vi "SMR_LabVIEW_V8.2.vi"() -> ()   [LabVIEW 2025]
uses:
  <vilib>/DAQmx/write.llb/DAQmx Write (Analog DBL 1Chan 1Samp).vi
  <vilib>/DAQmx/read.llb/DAQmx Read (Analog 1D DBL NChan 1Samp).vi
  <vilib>/DAQmx/read.llb/DAQmx Read (Analog 2D DBL NChan NSamp).vi
  <vilib>/Analysis/baseanly.llb/Mean (DBL).vi
  <vilib>/DAQmx/create/channels.llb/DAQmx Create Channel (AI-Temperature-Thermocouple).vi
  <vilib>/DAQmx/create/channels.llb/DAQmx Create Channel (AI-Voltage-Basic).vi
  <vilib>/DAQmx/create/channels.llb/DAQmx Create Channel (AO-Voltage-Basic).vi
  <vilib>/DAQmx/miscellaneous.llb/DAQmx Fill In Error Info.vi
  <vilib>/DAQmx/configure/timing.llb/DAQmx Timing (Sample Clock).vi
  <vilib>/addons/control/pid/pid.llb/PID (DBL).vi
  <vilib>/measure/maspectr.llb/FFT Power Spectrum and PSD for 1 Chan.vi
  <vilib>/measure/matone.llb/Extract Single Tone Information 1 Chan.vi
  <vilib>/addons/control/pid/NI_PID_pid.lvlib
  <vilib>/Analysis/NI_AALBase.lvlib
  <vilib>/ptbypt/NI_PtbyPt.lvlib
  <vilib>/measure/NI_MAPro.lvlib
panel:
  out "Rod Power (W)":dbl
  out "Current Through Rod (A)":dbl
  out "Time in Steady State (s)":dbl
  in  "Steady-State Dwell (s)":dbl
  out "Main Loop Flow (GPM)":dbl
  out "FM Amplitude":dbl
  out "FM Frequency":dbl
  out "Spectrum":cluster{"f0":dbl, "df":dbl, "magnitude":dbl[]}(graph)
  out "Raw Signal":waveform(dbl)(graph)
  out "Smoothed HX Flow (GPM)":dbl
  out "Flow History":dbl(graph)
  out "HX Flow (GPM)":dbl
  out "Voltage Across Rod (V)":dbl format="%0.2f"
  out "Current Run Folder":path
  in  "Log Root Folder":path=path "C:/Users/LocalUser/Documents/GitHub/thermal-loop/resources/v0.1.1/data/001"
  out "Raw NI9201 \nVoltage Display":T1
  in  "Loop Period (ms)":dbl=1000.0
  in  "Stop":bool
  out "Auto Steady State Threshold (deg C/min)":dbl
  out "Max dT/dt (deg C/min)":dbl
  out "Temp Change Rate (deg C/min)":dbl
  out "5-Min Baseline Complete":bool
  out "Rate Window Ready":bool
  out "Steady State":bool
  in  "Voltage Limit (V)":dbl=10.0
  in  "Temperature Limit (C)":dbl=50.0
  in  "Pressure Limit (psi)":dbl=15.0
  out "Max Voltage":bool
  out "Max Temperature":bool
  out "Max Pressure":bool
  out "Heat Exchanger Pressure History":dbl(graph)
  out "Main Loop Pressure History":T2(graph)
  out "Overall Avg Pressure (psi)":dbl
  out "Heat Exchanger Pressure P6 (psi)":dbl
  out "Main Loop Avg Pressure (psi)":dbl
  out "Pressure Display":T3
  out "Overall Pressure History":T4(graph)
  out "Max Loop Pressure (psi)":dbl
  out "Heat Exchanger Temperature History":cluster{"Waveform":dbl, "Waveform":dbl}(graph)
  out "Main Loop Temeperature History":T5(graph)
  out "Heat Exchanger Avg Temp (deg C)":dbl
  out "Temperature Display":T6
  out "Overall Temperature History":T7(graph)
  out "Overall Avg Temp (deg C)":dbl
  out "Max Loop Temp (deg C)":dbl
  out "Final P-Valve Voltage (V)":dbl
  out "PID Trim Voltage (V)":dbl
  in  "PID Temp Setpoint (deg C)":dbl
  in  "Auto PID Enable":bool
  in  "Manual P-Valve Voltage (V)":dbl min=0.0 max=10.0
  out "Main Loop Avg Temp (deg C)":dbl
  # "Heat Exchanger Flow"
  # "Control/Troubleshoot"
  # "Steady State"
  # "Emergency Indicators"
  # "Pressure"
  # "Temperature"
  # "Proportional Valve Control"
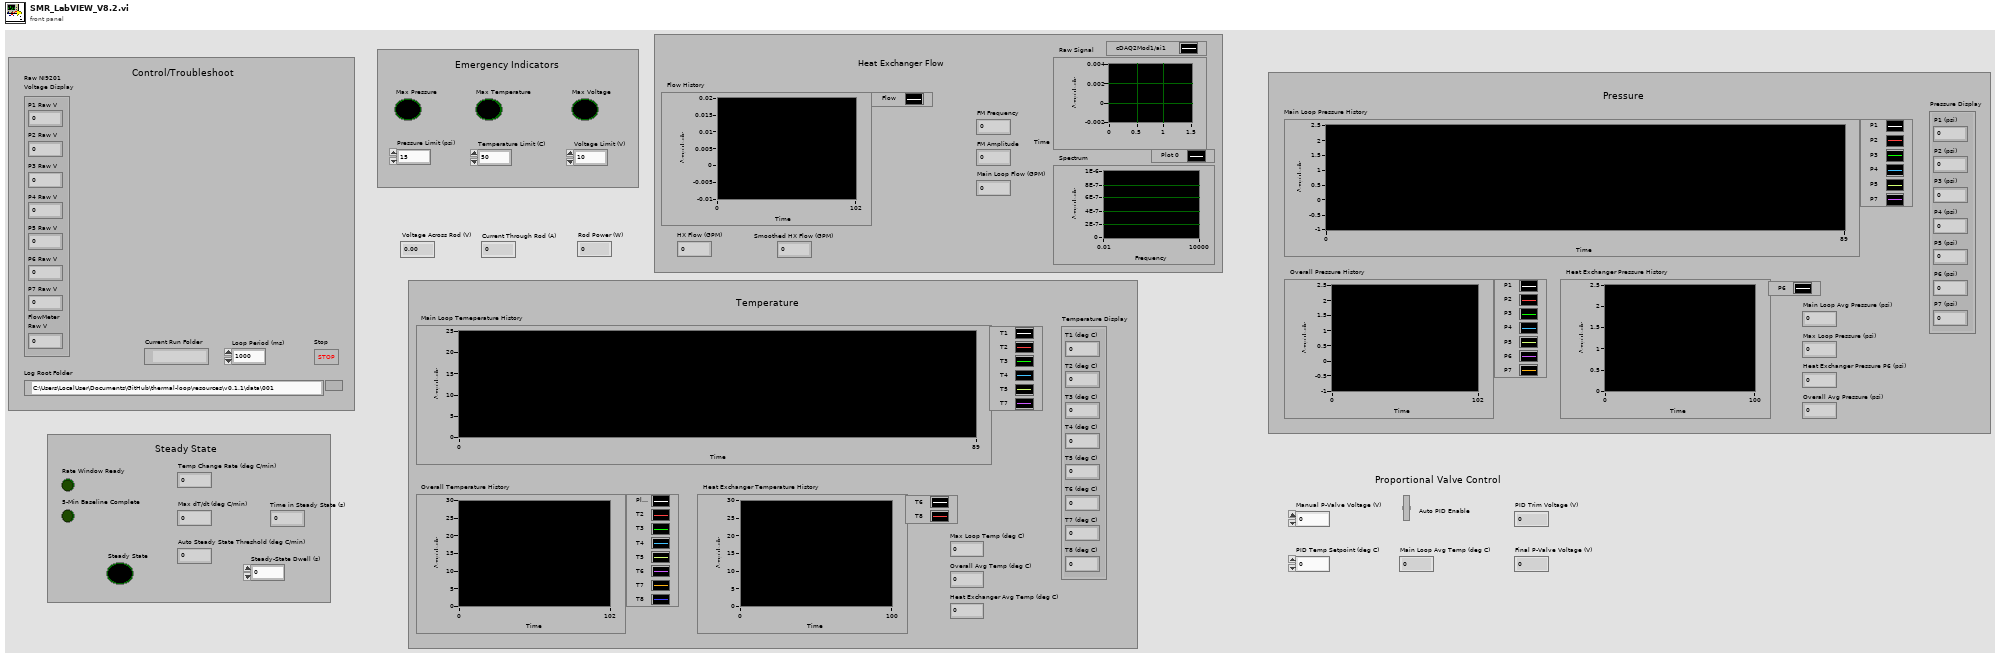
[diagram p1: front panel]
types:
  T1 = cluster{"P1 Raw V":dbl, "P2 Raw V":dbl, "P3 Raw V":dbl, "P4 Raw V":dbl, "P5 Raw V":dbl, "P6 Raw V":dbl, "P7 Raw V":dbl, "FlowMeter\nRaw V":dbl}
  T2 = cluster{"P1":dbl, "P2":dbl, "P3":dbl, "P4":dbl, "P5":dbl, "P7":dbl}
  T3 = cluster{"P1 (psi)":dbl, "P2 (psi)":dbl, "P3 (psi)":dbl, "P4 (psi)":dbl, "P5 (psi)":dbl, "P6 (psi)":dbl, "P7 (psi)":dbl}
  T4 = cluster{"P1":dbl, "P2":dbl, "P3":dbl, "P4":dbl, "P5":dbl, "P6":dbl, "P7":dbl}
  T5 = cluster{"Waveform":dbl, "Waveform":dbl, "Waveform":dbl, "Waveform":dbl, "Waveform":dbl, "Waveform":dbl}
  T6 = cluster{"T1 (deg C)":dbl, "T2 (deg C)":dbl, "T3 (deg C)":dbl, "T4 (deg C)":dbl, "T5 (deg C)":dbl, "T6 (deg C)":dbl, "T7 (deg C)":dbl, "T8 (deg C)":dbl}
  T7 = cluster{"Waveform":dbl, "Waveform":dbl, "Waveform":dbl, "Waveform":dbl, "Waveform":dbl, "Waveform":dbl, "Waveform":dbl, "Waveform":dbl}
  T8 = enum16{"open", "replace", "create", "open or create", "replace or create", "replace or create with confirmation"}
  T9 = cluster{"proportional gain (Kc)":dbl, "integral time (Ti, min)":dbl, "derivative time (Td, min)":dbl}
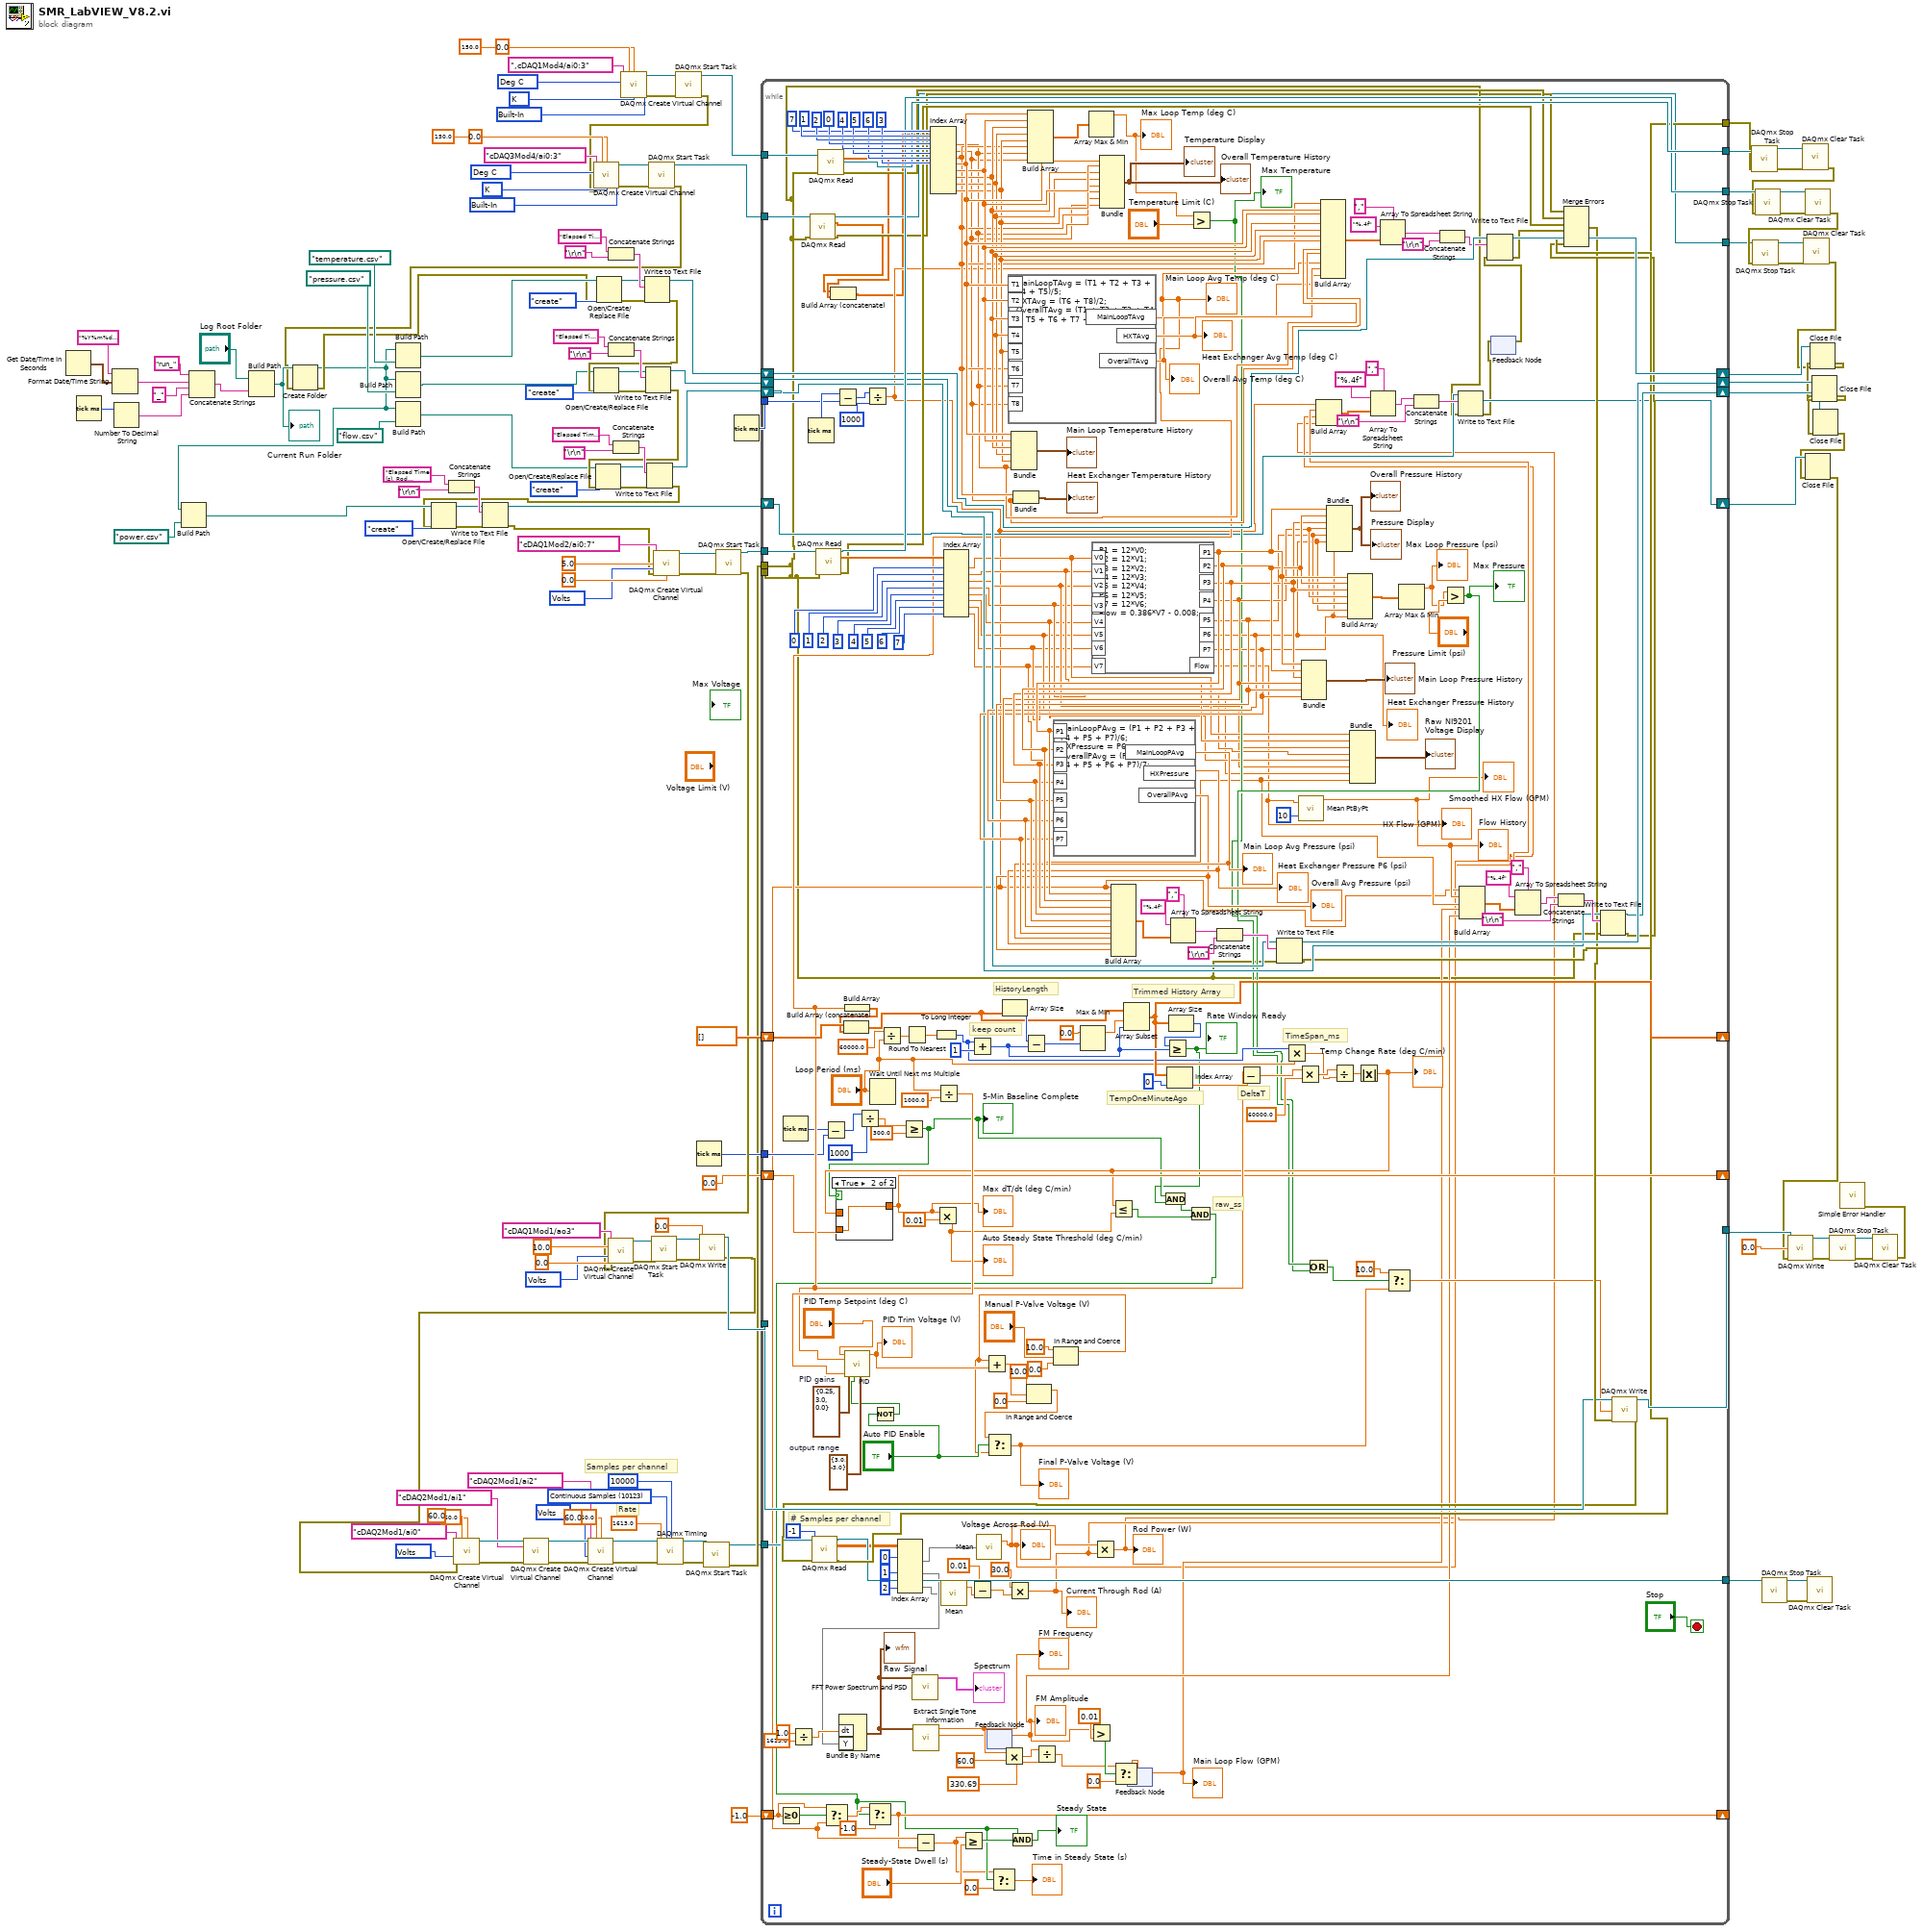
[diagram p0: block diagram]
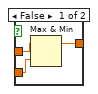
[diagram p2: hidden frame]
diagram:
  w3 = 10348 items=["Volts"=10348, "From Custom Scale"=10065] ("units")
  w20 = 10200 items=["Built-In"=10200, "Constant Value"=10116, "Channel"=10113] ("cjc source")
  w21 = 10073 items=["J"=10072, "K"=10073, "N"=10077, "R"=10082, "S"=10085, "T"=10086, "B"=10047, "E"=10055] ("thermocouple type")
  w22 = 10143 items=["Deg C"=10143, "Deg F"=10144, "Kelvins"=10325, "Deg R"=10145, "From Custom Scale"=10065] ("units")
  w53 = 10123 items=["Finite Samples"=10178, "Continuous Samples"=10123, "Hardware Timed Single Point"=12522] ("sample mode")
  w55 = 10348 items=["Volts"=10348, "From Custom Scale"=10065] ("units")
  w75 = 10348 items=["Volts"=10348, "From Custom Scale"=10065] ("units")
  w137 = 10200 items=["Built-In"=10200, "Constant Value"=10116, "Channel"=10113] ("cjc source")
  w138 = 10073 items=["J"=10072, "K"=10073, "N"=10077, "R"=10082, "S"=10085, "T"=10086, "B"=10047, "E"=10055] ("thermocouple type")
  w139 = 10143 items=["Deg C"=10143, "Deg F"=10144, "Kelvins"=10325, "Deg R"=10145, "From Custom Scale"=10065] ("units")
  w146 = 10348 items=["Volts"=10348, "From Custom Scale"=10065] ("units")
  # "Samples per channel"
  # "Rate"
  n1 = Get Date/Time In Seconds() -> (seconds since 1Jan1904=w96:timestamp)
  n2 = Tick Count (ms)() -> (millisecond timer value=w94:u32)
  n3 = Format Date/Time String(time format string (%c)="%Y%m%d_%H%M%S", seconds (now)=w96) -> (date/time string=w91:string)  [unwired: 1 in]
  n4 = Number To Decimal String(number=w94) -> (decimal integer string=w92:string)  [unwired: 1 in]
  n5 = Concatenate Strings("run_" ("string"), w91, "_" ("string"), w92) -> (w88:string)
  n6 = Build Path(base path="Log Root Folder", name or relative path=w88) -> (appended path=w87:path)
  "Current Run Folder" <- w87
  n7 = Concatenate Strings("Elapsed Time (s), Rod voltage (V), Rod Current (A), Rod Power (W)", "\r\n") -> (w39:string)
  n8 = Concatenate Strings("Elapsed Time (s),T1 (deg C),T2 (deg C),T3 (deg C),T4 (deg C),T5 (deg C),T6 (deg C),T7 (deg C),T8 (deg C),Main Loop Avg Temp (deg C),HX Avg Temp (deg C),Overall Avg Temp (deg C)", "\r\n") -> (w120:string)
  n9 = Concatenate Strings("Elapsed Time (s),P1 (psi),P2 (psi),P3 (psi),P4 (psi),P5 (psi),P6 (psi),P7 (psi),Main Loop Avg Pressure (psi),HX Pressure (psi),Overall Avg Pressure (psi)", "\r\n") -> (w118:string)
  n10 = Concatenate Strings("Elapsed Time (s),Heat Exchanger Flow (GPM),Flow Raw Voltage (V), Main Loop Flow (GPM), Flow Signal Amplitude (V)", "\r\n") -> (w114:string)
  n11 = call-poly <vilib>:"DAQmx Create Virtual Channel.vi"("maximum value"=150.0, "minimum value"=0.0, "physical channels"=tag ",cDAQ1Mod4/ai0:3", "cjc source"=w137, "units"=w139, "thermocouple type"=w138) -> ("task out"=w136:refnum<k21>, "error out"=w135:errorcluster)  [unwired: 8 in]
  n12 = call <vilib>:"DAQmx Start Task.vi"("task/channels in"=w136, "error in"=w135) -> ("task out"=w134:refnum<k21>, "error out"=w16:errorcluster)  [unwired: 12 in]
  n13 = call-poly <vilib>:"DAQmx Create Virtual Channel.vi"("maximum value"=150.0, "minimum value"=0.0, "physical channels"=tag "cDAQ3Mod4/ai0:3", "cjc source"=w20, "units"=w22, "error in"=w16, "thermocouple type"=w21) -> ("task out"=w19:refnum<k21>, "error out"=w18:errorcluster)  [unwired: 7 in]
  n14 = call <vilib>:"DAQmx Start Task.vi"("task/channels in"=w19, "error in"=w18) -> ("task out"=w14:refnum<k21>, "error out"=w15:errorcluster)  [unwired: 12 in]
  n15 = Create Folder(path (use dialog)=w87, error in=w15) -> (created path=w33:path, error out=w80:errorcluster)  [unwired: 1 in, 1 out]
  n16 = Build Path(base path=w33, name or relative path=path "power.csv") -> (appended path=w34:path)
  n17 = Build Path(base path=w33, name or relative path=path "temperature.csv") -> (appended path=w86:path)
  n18 = Build Path(base path=w33, name or relative path=path "pressure.csv") -> (appended path=w85:path)
  n19 = Build Path(base path=w33, name or relative path=path "flow.csv") -> (appended path=w84:path)
  n20 = Open/Create/Replace File(file path (use dialog)=w86, error in=w80, operation (0:open)=T8."create") -> (refnum out=w119:refnum<file>, error out=w103:errorcluster)  [unwired: 3 in, 1 out]
  n21 = Write to Text File(file (use dialog)=w119, text=w120, error in=w103) -> (refnum out=w110:refnum<file>, error out=w102:errorcluster)  [unwired: 1 in, 1 out]
  n22 = Open/Create/Replace File(file path (use dialog)=w85, error in=w102, operation (0:open)=T8."create") -> (refnum out=w117:refnum<file>, error out=w101:errorcluster)  [unwired: 3 in, 1 out]
  n23 = Write to Text File(file (use dialog)=w117, text=w118, error in=w101) -> (refnum out=w109:refnum<file>, error out=w100:errorcluster)  [unwired: 1 in, 1 out]
  n24 = Open/Create/Replace File(file path (use dialog)=w84, error in=w100, operation (0:open)=T8."create") -> (refnum out=w113:refnum<file>, error out=w99:errorcluster)  [unwired: 3 in, 1 out]
  n25 = Write to Text File(file (use dialog)=w113, text=w114, error in=w99) -> (refnum out=w108:refnum<file>, error out=w31:errorcluster)  [unwired: 1 in, 1 out]
  n26 = Open/Create/Replace File(file path (use dialog)=w34, error in=w31, operation (0:open)=T8."create") -> (refnum out=w38:refnum<file>, error out=w35:errorcluster)  [unwired: 3 in, 1 out]
  n27 = Write to Text File(file (use dialog)=w38, text=w39, error in=w35) -> (refnum out=w29:refnum<file>, error out=w30:errorcluster)  [unwired: 1 in, 1 out]
  n28 = call-poly <vilib>:"DAQmx Create Virtual Channel.vi"("maximum value"=5.0, "minimum value"=0.0, "physical channels"=tag "cDAQ1Mod2/ai0:7", "units"=w146, "error in"=w30) -> ("task out"=w145:refnum<k21>, "error out"=w144:errorcluster)  [unwired: 9 in]
  n29 = Tick Count (ms)() -> (millisecond timer value=w60:u32)
  n30 = call <vilib>:"DAQmx Start Task.vi"("task/channels in"=w145, "error in"=w144) -> ("task out"=w143:refnum<k21>, "error out"=w68:errorcluster)  [unwired: 12 in]
  n31 = call-poly <vilib>:"DAQmx Create Virtual Channel.vi"("maximum value"=10.0, "minimum value"=0.0, "physical channels"=tag "cDAQ1Mod1/ao3", "units"=w75, "error in"=w68) -> ("task out"=w74:refnum<k21>, "error out"=w73:errorcluster)  [unwired: 9 in]
  n32 = call <vilib>:"DAQmx Start Task.vi"("task/channels in"=w74, "error in"=w73) -> ("task out"=w72:refnum<k21>, "error out"=w71:errorcluster)  [unwired: 12 in]
  n33 = call-poly <vilib>:"DAQmx Write.vi"("task/channels in"=w72, "data"=0.0, "error in"=w71) -> ("task out"=w69:refnum<k21>, "error out"=w47:errorcluster)  [unwired: 10 in, 1 out]
  n34 = call-poly <vilib>:"DAQmx Create Virtual Channel.vi"("maximum value"=60.0, "minimum value"=-60.0, "physical channels"=tag "cDAQ2Mod1/ai0", "units"=w55, "error in"=w47) -> ("task out"=w43:refnum<k21>, "error out"=w42:errorcluster)  [unwired: 9 in]
  n35 = call-poly <vilib>:"DAQmx Create Virtual Channel.vi"("task in"=w43, "physical channels"=tag "cDAQ2Mod1/ai1", "error in"=w42) -> ("task out"=w7:refnum<k21>, "error out"=w5:errorcluster)  [unwired: 11 in]
  n36 = call-poly <vilib>:"DAQmx Create Virtual Channel.vi"("task in"=w7, "maximum value"=60.0, "minimum value"=-60.0, "physical channels"=tag "cDAQ2Mod1/ai2", "units"=w3, "error in"=w5) -> ("task out"=w6:refnum<k21>, "error out"=w4:errorcluster)  [unwired: 8 in]
  n37 = call-poly <vilib>:"DAQmx Timing.vi"("task/channels in"=w6, "sample mode"=w53, "samples per channel"=10000, "rate"=1613.0, "error in"=w4) -> ("task out"=w51:refnum<k21>, "error out"=w50:errorcluster)  [unwired: 9 in]
  n38 = call <vilib>:"DAQmx Start Task.vi"("task/channels in"=w51, "error in"=w50) -> ("task out"=w45:refnum<k21>, "error out"=w46:errorcluster)  [unwired: 12 in]
  n39 = Tick Count (ms)() -> (millisecond timer value=w107:u32)
  n40 = while {
    tunnel: w143 -> [w375]
    tunnel: w134 -> [w358]
    tunnel: [w349] -> w133
    tunnel: [w164] -> _
    tunnel: [w348] -> w132
    tunnel: [w224] -> w131
    shift-right: [w325] -> w106
    shift-left: w110 -> [w326]
    shift-right: [w306] -> w105
    shift-left: w109 -> [w307]
    shift-right: [w298] -> w104
    shift-left: w108 -> [w299]
    tunnel: w107 -> [w344]
    shift-right: [w277] -> _
    shift-left: dbl[] [] -> [w290]
    tunnel: w69 -> [w258]
    tunnel: w46 -> [w164]
    tunnel: [w265] -> w66
    tunnel: w60 -> [w247]
    shift-right: [w240] -> _
    shift-left: 0.0 -> [w242]
    tunnel: w45 -> [w223]
    tunnel: [w222] -> w44
    shift-right: [w181] -> w28
    shift-left: w29 -> [w182]
    shift-right: [w173] -> _
    shift-left: -1.0 -> [w177]
    tunnel: w14 -> [w165]
    tunnel: [w162] -> w10
    stop <- "Stop" stop-if-true
    w263 = cluster{"output high":dbl, "output low":dbl} {"output high"=3.0, "output low"=-3.0}  # output range
    w264 = T9 {"proportional gain (Kc)"=0.25, "integral time (Ti, min)"=3.0, "derivative time (Td, min)"=0.0}  # PID gains
    # "raw_ss"
    # "# Samples per channel"
    # "TimeSpan_ms"
    # "DeltaT"
    # "TempOneMinuteAgo"
    # "Trimmed History Array"
    # "HistoryLength"
    # "keep count"
    n41 = Greater Or Equal To 0?(x=w177) -> (x >= 0?=w178:bool)
    n42 = Tick Count (ms)() -> (millisecond timer value=w248:u32)
    n43 = Divide(x=1.0, y=1613.0) -> (x/y=w195:dbl)
    n44 = Tick Count (ms)() -> (millisecond timer value=w345:u32)
    n45 = call-poly <vilib>:"DAQmx Read.vi"("task/channels in"=w165, "error in"=w164) -> ("task out"=w162:refnum<k21>, "data"=w159:dbl[], "error out"=w163:errorcluster)  [unwired: 11 in]
    n46 = call-poly <vilib>:"DAQmx Read.vi"("task/channels in"=w375, "error in"=w164) -> ("task out"=w348:refnum<k21>, "data"=w366:dbl[], "error out"=w346:errorcluster)  [unwired: 11 in]
    n47 = call-poly <vilib>:"DAQmx Read.vi"("task/channels in"=w358, "error in"=w164) -> ("task out"=w349:refnum<k21>, "data"=w160:dbl[], "error out"=w347:errorcluster)  [unwired: 11 in]
    n48 = Subtract(x=w248, y=w247) -> (x-y=w246:u32)
    n49 = Build Array (concatenate)(w159, w160) -> (w161:dbl[])
    n50 = Subtract(x=w345, y=w344) -> (x-y=w343:u32)
    n51 = Divide(x=w246, y=u32 1000) -> (x/y=w244:dbl)
    n52 = Divide(x=w343, y=u32 1000) -> (x/y=w174:dbl)
    n53 = Select(t=w177, s=w178, f=w174) -> (s? t:f=w176:dbl)
    n54 = Wait Until Next ms Multiple(millisecond multiple="Loop Period (ms)") -> ()  [unwired: 1 out]
    n55 = Not(x="Auto PID Enable") -> (.not. x?=w259:bool)
    n56 = Divide(x=60000.0, y="Loop Period (ms)") -> (x/y=w287:dbl)
    n57 = Greater Or Equal?(x=w244, y=300.0) -> (x >= y?=w237:bool)
    "5-Min Baseline Complete" <- w237
    n58 = Round To Nearest(number=w287) -> (nearest integer value=w286:dbl)
    n59 = Index Array(array=w161, index #1=7 ("index"), index #2=1 ("index"), index #3=2 ("index"), index #4=0 ("index"), index #5=4 ("index"), index #6=5 ("index"), index #7=6 ("index"), index #8=3 ("index")) -> (element #1=w335:dbl, element #2=w334:dbl, element #3=w336:dbl, element #4=w341:dbl, element #5=w340:dbl, element #6=w339:dbl, element #7=w338:dbl, element #8=w337:dbl)
    n60 = To Long Integer(number=w286) -> (32bit integer=w274:i32)
    n61 = Divide(x="Loop Period (ms)", y=1000.0) -> (x/y=w260:dbl)
    n62 = Index Array(array=w366, index #1=0 ("index"), index #2=1 ("index"), index #3=2 ("index"), index #4=3 ("index"), index #5=4 ("index"), index #6=5 ("index"), index #7=6 ("index"), index #8=7 ("index")) -> (element #1=w221:dbl, element #2=w220:dbl, element #3=w219:dbl, element #4=w218:dbl, element #5=w217:dbl, element #6=w216:dbl, element #7=w215:dbl, element #8=w214:dbl)
    n63 = Add(x=w274, y=1) -> (x+y=w279:i32)
    n64 = feedback #1() -> (w191:dbl)  [unwired: 1 in]
    "FM Amplitude" <- w191
    n65 = formula code="MainLoopTAvg = (T1 + T2 + T3 + T4 + T5)/5;\nHXTAvg = (T6 + T8)/2;\nOverallTAvg = (T1 + T2 + T3 + T4 + T5 + T6 + T7 + T8)/8;"("T1"=w341, "T2"=w340, "T3"=w339, "T4"=w338, "T5"=w337, "T6"=w336, "T7"=w335, "T8"=w334) -> ("MainLoopTAvg"=w250:dbl, "HXTAvg"=w333:dbl, "OverallTAvg"=w332:dbl)
    "Overall Avg Temp (deg C)" <- w332
    "Main Loop Avg Temp (deg C)" <- w250
    "Heat Exchanger Avg Temp (deg C)" <- w333
    n66 = Build Array(w250) -> (w289:dbl[])
    n67 = Build Array (concatenate)(w290, w289) -> (w281:dbl[])
    n68 = call-poly <vilib>:"PID.vi"("reinitialize? (F)"=w259, "output range"=w263, "dt (s)"=w260, "PID gains"=w264, "process variable"=w250, "setpoint"="PID Temp Setpoint (deg C)") -> ("output"=w257:dbl)  [unwired: 4 in, 1 out]
    "PID Trim Voltage (V)" <- w257
    n69 = Array Size(array=w281) -> (size(s)=w284:i32)
    n70 = Bundle("Waveform"=w341, "Waveform"=w340, "Waveform"=w339, "Waveform"=w338, "Waveform"=w337, "Waveform"=w335) -> (→"Main Loop Temeperature History":T5)  [unwired: 1 in]
    n71 = Bundle("Waveform"=w336, "Waveform"=w334) -> (→"Heat Exchanger Temperature History":cluster{"Waveform":dbl, "Waveform":dbl})  [unwired: 1 in]
    n72 = Subtract(x=w284, y=w279) -> (x-y=w282:i32)
    n73 = Build Array(w341, w340, w339, w338, w337, w336, w335, w334) -> (w376:dbl[])
    n74 = In Range and Coerce(upper limit=10.0, x="Manual P-Valve Voltage (V)", lower limit=0.0) -> (coerced(x)=w252:dbl)  [unwired: 1 out]
    n75 = Add(x=w252, y=w257) -> (x+y=w256:dbl)
    n76 = In Range and Coerce(upper limit=10.0, x=w256, lower limit=0.0) -> (coerced(x)=w251:dbl)  [unwired: 1 out]
    n77 = Select(t=w251, s="Auto PID Enable", f=w252) -> (s? t:f=w229:dbl)
    "Final P-Valve Voltage (V)" <- w229
    n78 = Max & Min(x=0.0, y=w282) -> (max(x,y)=w280:dbl)  [unwired: 1 out]
    n79 = Array Max & Min(array=w376) -> (max value=w292:dbl)  [unwired: 3 out]
    "Max Loop Temp (deg C)" <- w292
    n80 = Greater?(x=w191, y=0.01) -> (0:w199:bool)
    n81 = formula code="P1 = 12*V0;\nP2 = 12*V1;\nP3 = 12*V2;\nP4 = 12*V3;\nP5 = 12*V4;\nP6 = 12*V5; \nP7 = 12*V6;\nFlow = 0.386*V7 - 0.008;"("V0"=w221, "V1"=w220, "V2"=w219, "V3"=w218, "V4"=w217, "V5"=w216, "V6"=w215, "V7"=w214) -> ("P1"=w324:dbl, "P2"=w323:dbl, "P3"=w322:dbl, "P4"=w321:dbl, "P5"=w320:dbl, "P6"=w319:dbl, "P7"=w318:dbl, "Flow"=w213:dbl)
    "HX Flow (GPM)" <- w213
    "Heat Exchanger Pressure History" <- w319
    n82 = formula code="MainLoopPAvg = (P1 + P2 + P3 + P4 + P5 + P7)/6;\nHXPressure = P6;\nOverallPAvg = (P1 + P2 + P3 + P4 + P5 + P6 + P7)/7;"("P1"=w324, "P2"=w323, "P3"=w322, "P4"=w321, "P5"=w320, "P6"=w319, "P7"=w318) -> ("MainLoopPAvg"=w317:dbl, "HXPressure"=w316:dbl, "OverallPAvg"=w315:dbl)
    "Overall Avg Pressure (psi)" <- w315
    "Heat Exchanger Pressure P6 (psi)" <- w316
    "Main Loop Avg Pressure (psi)" <- w317
    n83 = Bundle("Waveform"=w341, "Waveform"=w340, "Waveform"=w339, "Waveform"=w338, "Waveform"=w337, "Waveform"=w336, "Waveform"=w335, "Waveform"=w334) -> (→"Overall Temperature History" →"Temperature Display":T7)  [unwired: 1 in]
    n84 = Build Array(w174, w324, w323, w322, w321, w320, w319, w318, w317, w316, w315) -> (w314:dbl[])
    n85 = Array Subset(array=w281, index=w280, length=w279) -> (w277:dbl[])
    n86 = feedback #2() -> (w189:dbl)  [unwired: 1 in]
    "Main Loop Flow (GPM)" <- w189
    n87 = Index Array(array=w277, index=0) -> (element=w275:dbl)
    n88 = Array Size(array=w277) -> (size(s)=w278:i32)
    n89 = Greater Or Equal?(x=w278, y=w279) -> (x >= y?=w236:bool)
    "Rate Window Ready" <- w236
    n90 = And(x=w237, y=w236) -> (x .and. y?=w235:bool)
    n91 = Array To Spreadsheet String(delimiter (Tab)=",", array=w314, 3:"%.4f" ("format string")) -> (spreadsheet string=w310:string)
    n92 = Greater?(x=w292, y="Temperature Limit (C)") -> (0:w232:bool)
    "Max Temperature" <- w232
    n93 = Concatenate Strings(w310, "\r\n") -> (w308:string)
    n94 = Subtract(x=w250, y=w275) -> (x-y=w273:dbl)
    n95 = Write to Text File(file (use dialog)=w307, text=w308, error in=w164) -> (refnum out=w306:refnum<file>, error out=w296:errorcluster)  [unwired: 1 in, 1 out]
    n96 = Multiply(x=w274, y="Loop Period (ms)") -> (x*y=w270:dbl)
    n97 = Multiply(x=w273, y=60000.0) -> (x*y=w271:dbl)
    n98 = call <vilib>:"Mean PtByPt.vi"("x"=w213, "sample length"=10) -> ("mean"=w211:dbl)  [unwired: 2 in, 1 out]
    "Flow History" <- w211
    "Smoothed HX Flow (GPM)" <- w211
    n99 = Bundle("P1"=w324, "P2"=w323, "P3"=w322, "P4"=w321, "P5"=w320, "P7"=w318) -> (→"Main Loop Pressure History":T2)  [unwired: 1 in]
    n100 = Build Array(w174, w341, w340, w339, w338, w337, w336, w335, w334, w250, w333, w332) -> (w331:dbl[])
    n101 = Bundle("P1"=w324, "P2"=w323, "P3"=w322, "P4"=w321, "P5"=w320, "P6"=w319, "P7"=w318) -> (→"Overall Pressure History" →"Pressure Display":T4)  [unwired: 1 in]
    n102 = Divide(x=w271, y=w270) -> (x/y=w269:dbl)
    n103 = Build Array(w324, w323, w322, w321, w320, w319, w318) -> (w365:dbl[])
    n104 = Bundle("Waveform"=w221, "Waveform"=w220, "Waveform"=w219, "Waveform"=w218, "Waveform"=w217, "Waveform"=w216, "Waveform"=w215, "Waveform"=w214) -> (→"Raw NI9201 \nVoltage Display":T7)  [unwired: 1 in]
    n105 = Absolute Value(x=w269) -> (abs(x)=w239:dbl)
    "Temp Change Rate (deg C/min)" <- w239
    n106 = case shown="True" w237 {
      tunnel: w242 -> [w380 w381]
      tunnel: w239 -> [w379 _]
      tunnel: [w378 w381] -> w240
      frame False {
        n107 = Max & Min(x=w379, y=w380) -> (max(x,y)=w378:dbl)  [unwired: 1 out]
      }
      frame True {
      }
    }
    "Max dT/dt (deg C/min)" <- w240
    n108 = Multiply(x=w240, y=0.01) -> (x*y=w238:dbl)
    "Auto Steady State Threshold (deg C/min)" <- w238
    n109 = Less Or Equal?(x=w239, y=w238) -> (x <= y?=w234:bool)
    n110 = And(x=w235, y=w234) -> (x .and. y?=w169:bool)
    n111 = Select(t=w176, s=w169, f=-1.0) -> (s? t:f=w173:dbl)
    n112 = Subtract(x=w174, y=w173) -> (x-y=w168:dbl)
    n113 = Greater Or Equal?(x=w168, y="Steady-State Dwell (s)") -> (x >= y?=w171:bool)
    n114 = Select(t=w168, s=w169, f=0.0) -> (s? t:f=→"Time in Steady State (s)":dbl)
    n115 = And(x=w169, y=w171) -> (x .and. y?=→"Steady State":bool)
    n116 = Array To Spreadsheet String(delimiter (Tab)=",", array=w331, 3:"%.4f" ("format string")) -> (spreadsheet string=w328:string)
    n117 = Array Max & Min(array=w365) -> (max value=w293:dbl)  [unwired: 3 out]
    "Max Loop Pressure (psi)" <- w293
    n118 = Concatenate Strings(w328, "\r\n") -> (w311:string)
    n119 = Greater?(x=w293, y="Pressure Limit (psi)") -> (0:w233:bool)
    "Max Pressure" <- w233
    n120 = Or(x=w233, y=w232) -> (x .or. y?=w227:bool)
    n121 = Select(t=10.0, s=w227, f=w229) -> (s? t:f=w228:dbl)
    n122 = Build Array(w174, w211, w214, w189, w191) -> (w305:dbl[])
    n123 = feedback #3() -> (w179:errorcluster)  [unwired: 1 in]
    n124 = Write to Text File(file (use dialog)=w326, text=w311, error in=w179) -> (refnum out=w325:refnum<file>, error out=w297:errorcluster)  [unwired: 1 in, 1 out]
    n125 = Array To Spreadsheet String(delimiter (Tab)=",", array=w305, 3:"%.4f" ("format string")) -> (spreadsheet string=w301:string)
    n126 = Concatenate Strings(w301, "\r\n") -> (w300:string)
    n127 = Write to Text File(file (use dialog)=w299, text=w300, error in=w164) -> (refnum out=w298:refnum<file>, error out=w295:errorcluster)  [unwired: 1 in, 1 out]
    n128 = Merge Errors(w163, w347, w346, w297, w296, w295) -> (w266:errorcluster)
    n129 = call-poly <vilib>:"DAQmx Write.vi"("task/channels in"=w258, "data"=w228, "error in"=w266) -> ("task out"=w265:refnum<k21>, "error out"=w225:errorcluster)  [unwired: 10 in, 1 out]
    n130 = call-poly <vilib>:"DAQmx Read.vi"("task/channels in"=w223, "number of samples per channel"=-1, "error in"=w225) -> ("task out"=w222:refnum<k21>, "data"=w210:dbl[][], "error out"=w224:errorcluster)  [unwired: 10 in]
    n131 = Index Array(array=w210, index (row) #1=0 ("index (row)"), index (row) #2=1 ("index (row)"), index (row) #3=2 ("index (row)")) -> (element #1=w209:dbl[], element #2=w194:dbl[], element #3=w154:dbl[])  [unwired: 3 in]
    n132 = Bundle By Name("dt"=w195, "Y"=w194) -> (w193:waveform(dbl))  [unwired: 1 in]
    "Raw Signal" <- w193
    n133 = call-poly <vilib>:"FFT Power Spectrum and PSD.vi"("time signal"=w193) -> ("Power Spectrum / PSD"=→"Spectrum":cluster{"f0":dbl, "df":dbl, "magnitude":dbl[]})  [unwired: 7 in, 3 out]
    n134 = call-poly <vilib>:"Extract Single Tone Information.vi"("time signal in"=w193) -> ("detected amplitude"=w192:dbl, "detected frequency"=w205:dbl)  [unwired: 5 in, 4 out]
    "FM Frequency" <- w205
    n135 = call-poly <vilib>:"Mean.vi"("X"=w154) -> ("mean"=w155:dbl)  [unwired: 1 out]
    n136 = Subtract(x=0.01, y=w155) -> (x-y=w156:dbl)
    n137 = call-poly <vilib>:"Mean.vi"("X"=w209) -> ("mean"=w152:dbl)  [unwired: 1 out]
    "Voltage Across Rod (V)" <- w152
    n138 = feedback-in #1(w192) -> ()
    n139 = Multiply(x=w205, y=60.0) -> (x*y=w203:dbl)
    n140 = Multiply(x=30.0, y=w156) -> (x*y=w151:dbl)
    "Current Through Rod (A)" <- w151
    n141 = Divide(x=w203, y=330.69) -> (x/y=w198:dbl)
    n142 = Multiply(x=w152, y=w151) -> (x*y=w150:dbl)
    "Rod Power (W)" <- w150
    n143 = Select(t=w198, s=w199, f=0.0) -> (s? t:f=w190:dbl)
    n144 = feedback-in #2(w190) -> ()
    n145 = Build Array(w174, w152, w151, w150) -> (w184:dbl[])
    n146 = Array To Spreadsheet String(delimiter (Tab)=",", array=w184, 3:"%.4f" ("format string")) -> (spreadsheet string=w187:string)
    n147 = Concatenate Strings(w187, "\r\n") -> (w183:string)
    n148 = Write to Text File(file (use dialog)=w182, text=w183, error in=w164) -> (refnum out=w181:refnum<file>, error out=w180:errorcluster)  [unwired: 1 in, 1 out]
    n149 = feedback-in #3(w180) -> ()
  }
  n150 = call <vilib>:"DAQmx Stop Task.vi"("task/channels in"=w133, "error in"=w131) -> ("task out"=w130:refnum<k21>, "error out"=w128:errorcluster)  [unwired: 12 in]
  n151 = call <vilib>:"DAQmx Stop Task.vi"("task/channels in"=w44) -> ("task out"=w49:refnum<k21>, "error out"=w48:errorcluster)  [unwired: 13 in]
  n152 = call <vilib>:"DAQmx Clear Task.vi"("task in"=w130, "error in"=w128) -> ("error out"=w127:errorcluster)  [unwired: 13 in]
  n153 = call <vilib>:"DAQmx Stop Task.vi"("task/channels in"=w132, "error in"=w127) -> ("task out"=w129:refnum<k21>, "error out"=w126:errorcluster)  [unwired: 12 in]
  n154 = call <vilib>:"DAQmx Clear Task.vi"("task in"=w129, "error in"=w126) -> ("error out"=w13:errorcluster)  [unwired: 13 in]
  n155 = call <vilib>:"DAQmx Stop Task.vi"("task/channels in"=w10, "error in"=w13) -> ("task out"=w9:refnum<k21>, "error out"=w12:errorcluster)  [unwired: 12 in]
  n156 = call <vilib>:"DAQmx Clear Task.vi"("task in"=w9, "error in"=w12) -> ("error out"=w11:errorcluster)  [unwired: 13 in]
  n157 = call <vilib>:"DAQmx Clear Task.vi"("task in"=w49, "error in"=w48) -> ()  [unwired: 13 in, 1 out]
  n158 = Close File(refnum=w106, error in=w11) -> (error out=w98:errorcluster)  [unwired: 1 out]
  n159 = Close File(refnum=w105, error in=w98) -> (error out=w97:errorcluster)  [unwired: 1 out]
  n160 = Close File(refnum=w104, error in=w97) -> (error out=w27:errorcluster)  [unwired: 1 out]
  n161 = Close File(refnum=w28, error in=w27) -> (error out=w26:errorcluster)  [unwired: 1 out]
  n162 = call-poly <vilib>:"DAQmx Write.vi"("task/channels in"=w66, "data"=0.0, "error in"=w26) -> ("task out"=w65:refnum<k21>, "error out"=w63:errorcluster)  [unwired: 10 in, 1 out]
  n163 = call <vilib>:"DAQmx Stop Task.vi"("task/channels in"=w65, "error in"=w63) -> ("task out"=w64:refnum<k21>, "error out"=w62:errorcluster)  [unwired: 12 in]
  n164 = call <vilib>:"DAQmx Clear Task.vi"("task in"=w64, "error in"=w62) -> ("error out"=w61:errorcluster)  [unwired: 13 in]
  n165 = call <vilib>:"Simple Error Handler.vi"("error in (no error)"=w61) -> ()  [unwired: 4 in, 5 out]
